vi "ExSubCreateImageDisplay.vi"(0 "Camera Handle":u32, 1 "Pulser Handle":u32, 2 "File and Display Name":string, 3 "error in (no error)":errorcluster) -> (5 "Handles Out":T1, 7 "error out":errorcluster)   [LabVIEW 2010]
panel:
  # "ExSubCreateFileMultImage.vi:\nThis is a SubVI that creates a file,  and image objects and returns the handles bundled in a cluster that includes a pulser and camera handle"
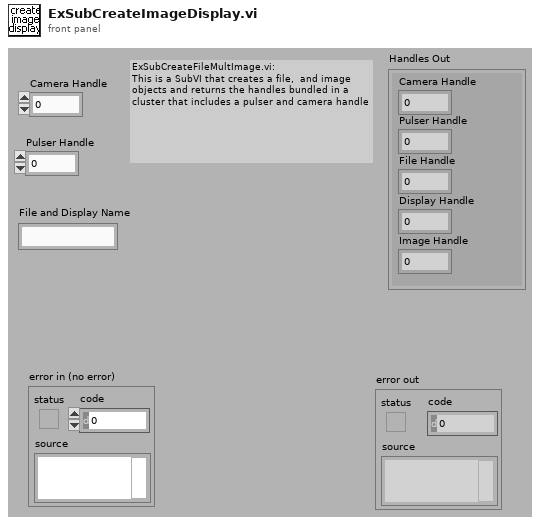
[diagram p1: front panel]
types:
  T1 = cluster{"Camera Handle":u32, "Pulser Handle":u32, "File Handle":u32, "Display Handle":u32, "Image Handle":u32}
  T2 = cluster{"Camera Handle":u32, "Pulser Handle":u32, i32, "Display Handle":u32, "Image Handle":u32}
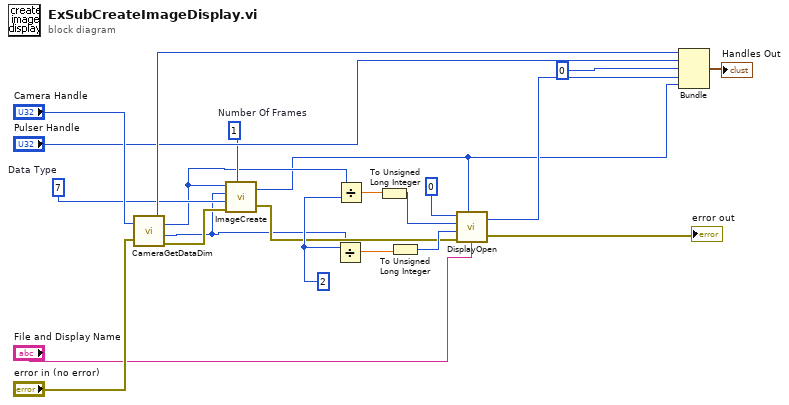
[diagram p0: block diagram]
diagram:
  w6 = u32 7  # Data Type
  w7 = u32 1  # Number Of Frames
  w13 = 2
  n1 = call <userlib>:"CameraGetDataDim.vi"("Camera Handle"="Camera Handle", "error in"="error in (no error)") -> ("Camera Handle"=w20:u32, "Xdim"=w5:u32, "Ydim"=w4:u32, "error out"=w9:errorcluster)
  n2 = call <userlib>:"ImageCreate.vi"("X dimension"=w5, "Y dimension"=w4, "Data Type"=w6, "error in"=w9, "Number Of Frames"=w7) -> ("Image Handle"=w1:u32, "error out"=w8:errorcluster)
  n3 = Divide(x=w4, y=w13) -> (x/y=w15:dbl)
  n4 = Divide(x=w5, y=w13) -> (x/y=w12:dbl)
  n5 = To Unsigned Long Integer(number=w12) -> (unsigned 32bit integer=w11:u32)
  n6 = To Unsigned Long Integer(number=w15) -> (unsigned 32bit integer=w14:u32)
  n7 = call <userlib>:"DisplayOpen.vi"("Display Title"="File and Display Name", "Image Handle"=w1, "error in"=w8, "Display Height"=w14, "Display Width"=w11, "Display Type"=0) -> ("error out"=→"error out":errorcluster, "Display Handle"=w18:u32)
  n8 = Bundle("Camera Handle"=w20, "Pulser Handle"="Pulser Handle", 0, "Display Handle"=w18, "Image Handle"=w1) -> (→"Handles Out":T2)  [unwired: 1 in]
